vi "1 channel N sample API.vi"() -> ()   [LabVIEW 2020]
uses:
  <vilib>/DAQmx/read.llb/DAQmx Read (Analog 1D DBL 1Chan NSamp).vi
  <vilib>/DAQmx/create/channels.llb/DAQmx Create Channel (AI-Temperature-Thermocouple).vi
  <vilib>/DAQmx/configure/timing.llb/DAQmx Timing (Sample Clock).vi
  <vilib>/DAQmx/miscellaneous.llb/DAQmx Fill In Error Info.vi
panel:
  out "Waveform Graph":dbl[](graph)
  in  "number of samples per channel( user defined to read from the daq)":i32=-1
  out "Array":dbl[](array[numeric]) format="%0.2f"
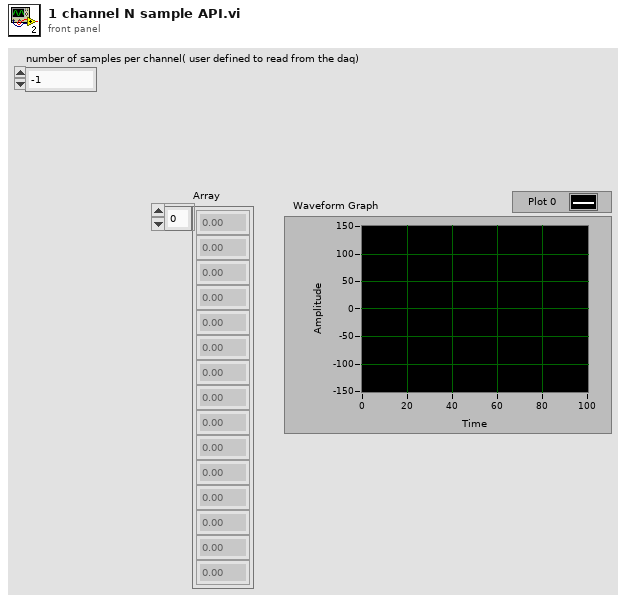
[diagram p1: front panel]
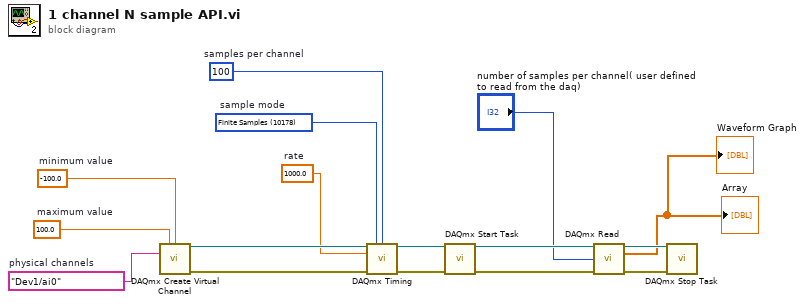
[diagram p0: block diagram]
diagram:
  w3 = 1000.0  # rate
  w6 = 10178 items=["Finite Samples"=10178, "Continuous Samples"=10123, "Hardware Timed Single Point"=12522]  # sample mode
  w7 = 100  # samples per channel
  w8 = 100.0  # maximum value
  w9 = -100.0  # minimum value
  w10 = tag "Dev1/ai0"  # physical channels
  n1 = call-poly <vilib>:"DAQmx Create Virtual Channel.vi"("maximum value"=w8, "minimum value"=w9, "physical channels"=w10) -> ("task out"=w5:refnum<k21>, "error out"=w14:errorcluster)  [unwired: 11 in]
  n2 = call-poly <vilib>:"DAQmx Timing.vi"("task/channels in"=w5, "sample mode"=w6, "samples per channel"=w7, "rate"=w3, "error in"=w14) -> ("task out"=w4:refnum<k21>, "error out"=w13:errorcluster)  [unwired: 9 in]
  n3 = call <vilib>:"DAQmx Start Task.vi"("task/channels in"=w4, "error in"=w13) -> ("task out"=w16:refnum<k21>, "error out"=w12:errorcluster)  [unwired: 12 in]
  n4 = call-poly <vilib>:"DAQmx Read.vi"("task/channels in"=w16, "number of samples per channel"="number of samples per channel( user defined to read from the daq)", "error in"=w12) -> ("task out"=w15:refnum<k21>, "data"=→"Array" →"Waveform Graph":dbl[], "error out"=w11:errorcluster)  [unwired: 10 in]
  n5 = call <vilib>:"DAQmx Stop Task.vi"("task/channels in"=w15, "error in"=w11) -> ()  [unwired: 12 in, 2 out]
